vi "write sys config device object.vi"(8 "error in":errorcluster, 10 "device information":T1 {"product ID" format="%.0x"}, 11 "syscfg device in":refnum<class "SysCfg Device.lvclass">) -> (0 "error out":errorcluster, 3 "syscfg device out":refnum<class "SysCfg Device.lvclass">)   [LabVIEW 2013, in "SMI.lvlib" / "SysCfg Device.lvclass"]
uses:
  SysCfg Device.lvclass
  sys config device information.ctl
  write system session.vi
  Device/write vendor name.vi
  Device/write product name.vi
  Device/write product ID.vi
  Device/write serial number.vi
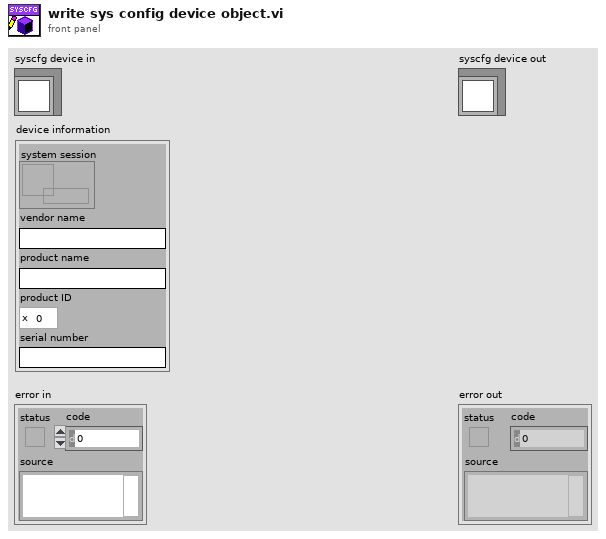
[diagram p1: front panel]
types:
  T1 = typedef "SMI.lvlib/SysCfg Device.lvclass/sys config device information.ctl" = cluster{"system session":refnum<data-value>, "vendor name":string, "product name":string, "product ID":u32, "serial number":string}
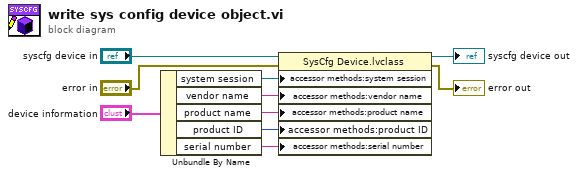
[diagram p0: block diagram]
diagram:
  n1 = Unbundle By Name("device information") -> ("system session"=w7:refnum<data-value>, "vendor name"=w6:string, "product name"=w5:string, "product ID"=w4:u32, "serial number"=w3:string)
  n2 = property class="SysCfg Device.lvclass"(reference="syscfg device in", error in="error in", "accessor methods:system session"=w7, "accessor methods:vendor name"=w6, "accessor methods:product name"=w5, "accessor methods:product ID"=w4, "accessor methods:serial number"=w3) -> (reference out=→"syscfg device out":refnum<class "SysCfg Device.lvclass">, error out=→"error out":errorcluster)
